vi "formula node.vi"() -> ()   [LabVIEW 2016]
panel:
  out "Waveform Graph":dbl[](graph)
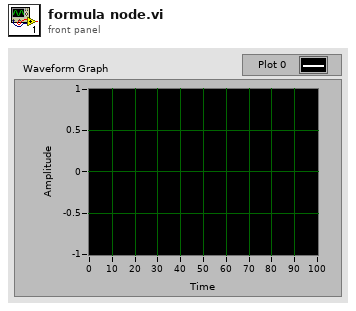
[diagram p1: front panel]
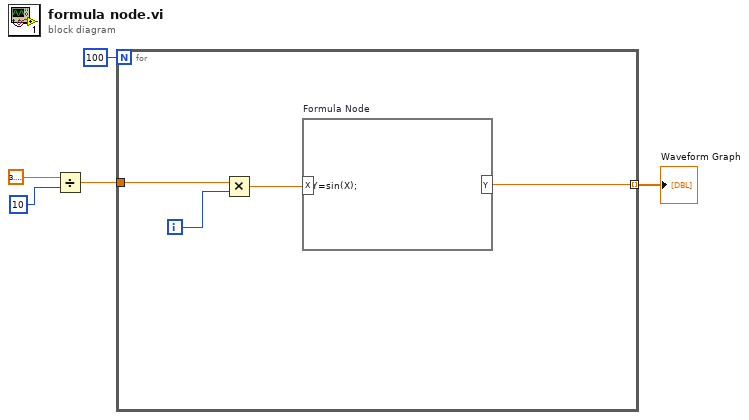
[diagram p0: block diagram]
diagram:
  n1 = Divide(x=3.141592653589793, y=10) -> (x/y=w2:dbl)
  n2 = for {
    N: 100 -> [_]
    tunnel: w2 -> [w9]
    tunnel: [w6] -> w1 mode=indexing
    i -> [w8]
    n3 = Multiply(x=w9, y=w8) -> (x*y=w7:dbl)
    n4 = formula code="Y=sin(X);"("X"=w7) -> ("Y"=w6:dbl)
  }
  "Waveform Graph" <- w1
